vi "Null Broadcast Events--constant.vi"() -> (3 "TCP-IP Engine Broadcast Events":T1)   [LabVIEW 2018, in "TCP-IP Engine.lvlib"]
doc: "Returns the broadcast events cluster with null references for defining the event types in a Register For Events function.\n_____\nBased on DQMH Project Template 7.0.1.1316."
uses:
  TCP-IP Engine.lvlib
  Broadcast Events--cluster.ctl
  Did Init Argument--cluster.ctl
  Status Updated Argument--cluster.ctl
  Error Reported Argument--cluster.ctl
  Stop Argument--cluster.ctl
  Get Module Execution Status Argument--cluster.ctl
  Open Connection Status Argument--cluster.ctl
  TCP-Read Data Out Argument--cluster.ctl
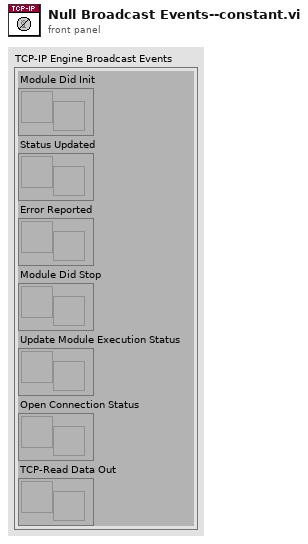
[diagram p1: front panel]
types:
  T1 = typedef "TCP-IP Engine.lvlib/Broadcast Events--cluster.ctl" = cluster{"Module Did Init":refnum<user-event>, "Status Updated":refnum<user-event>, "Error Reported":refnum<user-event>, "Module Did Stop":refnum<user-event>, "Update Module Execution Status":refnum<user-event>, "Open Connection Status":refnum<user-event>, "TCP-Read Data Out":refnum<user-event>}
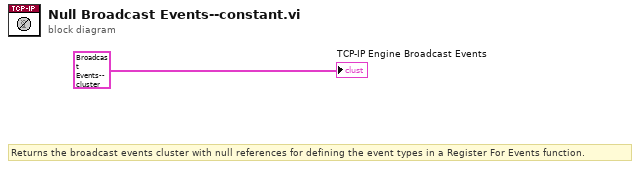
[diagram p0: block diagram]
diagram:
  # "Returns the broadcast events cluster with null references for defining the event types in a Register For Events function."
  "TCP-IP Engine Broadcast Events" <- T1 {"Module Did Init"=refnum, "Status Updated"=refnum, "Error Reported"=refnum, "Module Did Stop"=refnum, "Update Module Execution Status"=refnum, "Open Connection Status"=refnum, "TCP-Read Data Out"=refnum} ("Broadcast Events")
